vi "Upload File to Azure Container.vi"() -> ()   [LabVIEW 2015]
doc: "Demonstrates how to upload a file to an Azure Blob Service container."
uses:
  Core/Azure Credentials.ctl
  Blob Storage/Blob Type.ctl
  Core/NI_Azure_Core.lvlib
  Core/Session/Session.lvclass
  Blob Storage/NI_Azure_Blob.lvlib
panel:
  in  "File to Upload":path
  in  "Access Key":string
  in  "Storage Account Name":string
  in  "Destination Container":string
  # "Overview: Demonstrates how to upload a file to an Azure Blob Service container.\nRequirements: NI Cloud Toolkit for Azure and a registered Microsoft Azure account\nInstructions:\n1. Specify the Storage Account Name and Access Key for your Azure account. You can create an account at http://azure.microsoft.com.\n2. Specify a Destination Container for the file. If you have not created a container, you can run the Create New Azure Container.vi example to create a new container.\n3. Specify the File to Upload.\n4. Run the VI. The specified file will be placed in the specified container."
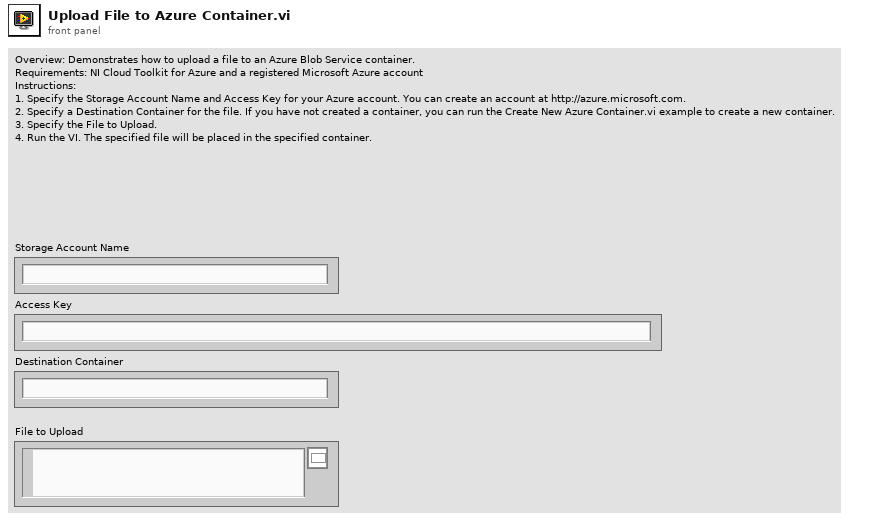
[diagram p1: front panel]
types:
  T1 = typedef "NI_Azure_Core.lvlib/Azure Credentials.ctl" = cluster{"Storage Account Name":string, "Access Key":string}
  T2 = typedef "NI_Azure_Blob.lvlib/Blob Type.ctl" = enum16{"BlockBlob", "PageBlob", "AppendBlob"}
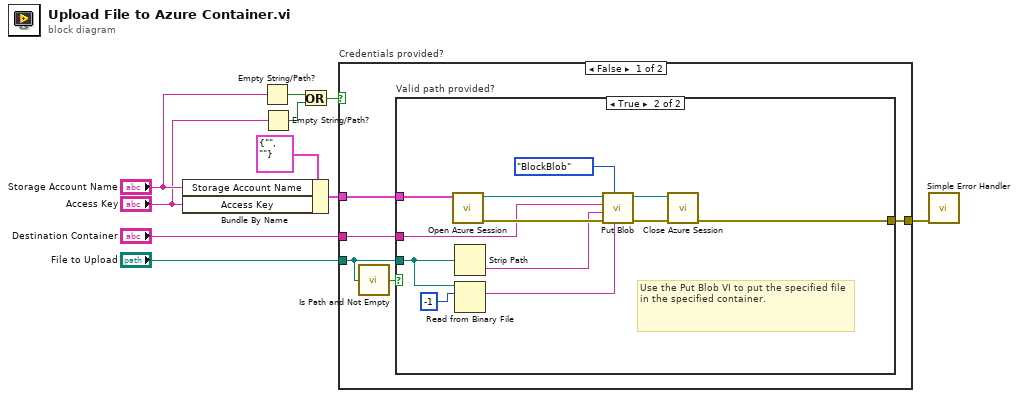
[diagram p0: block diagram]
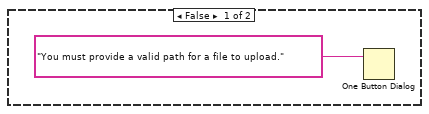
[diagram p2: hidden frame]
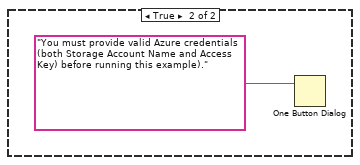
[diagram p3: hidden frame]
diagram:
  n1 = Bundle By Name(cluster=T1 {"Storage Account Name"="", "Access Key"=""} ("Credentials"), "Storage Account Name"="Storage Account Name", "Access Key"="Access Key") -> (w5:T1)
  n2 = Empty String/Path?(string/path="Storage Account Name") -> (empty?=w9:bool)
  n3 = Empty String/Path?(string/path="Access Key") -> (empty?=w10:bool)
  n4 = Or(x=w9, y=w10) -> (x .or. y?=w6:bool)
  n5 = case "Credentials provided?" shown="False" w6 {
    tunnel: w5 -> [w15 _]
    tunnel: "File to Upload" -> [w14 _]
    tunnel: "Destination Container" -> [w12 _]
    tunnel: [w11 _] -> w1
    frame False {
      n6 = call <vilib>:"Is Path and Not Empty.vi"("path"=w14) -> ("Is Path and Not Empty?"=w13:bool)  [unwired: 4 in]
      n7 = case "Valid path provided?" shown="True" w13 {
        tunnel: w15 -> [_ w28]
        tunnel: w14 -> [_ w24]
        tunnel: w12 -> [_ w19]
        tunnel: [_ w23] -> w11
        frame False {
          n8 = One Button Dialog(message="You must provide a valid path for a file to upload.") -> ()  [unwired: 1 in, 1 out]
        }
        frame True {
          # "Use the Put Blob VI to put the specified file in the specified container."
          n9 = call "Open Azure Session.vi"("Credentials"=w28) -> ("error out"=w27:errorcluster, "Azure Session"=w26:refnum<class "Session.lvclass">)  [unwired: 9 in]
          n10 = Strip Path(path=w24) -> (name=w18:string)  [unwired: 1 out]
          n11 = Read from Binary File(10:-1 ("count (1)"), 11:w24) -> (2:w21:string)  [unwired: 4 in, 3 out]
          n12 = call "Put Blob.vi"("Blob Content"=w21, "Blob type"=Blob_Type."BlockBlob", "error in (no error)"=w27, "Blob"=w18, "Container"=w19, "Azure Session in"=w26) -> ("error out"=w20:errorcluster, "Azure Session out"=w17:refnum<class "Session.lvclass">)  [unwired: 4 in]
          n13 = call "Close Azure Session.vi"("error in (no error)"=w20, "Azure Session"=w17) -> ("error out"=w23:errorcluster)  [unwired: 9 in]
        }
      }
    }
    frame True {
      n14 = One Button Dialog(message="You must provide valid Azure credentials (both Storage Account Name and Access Key) before running this example).") -> ()  [unwired: 1 in, 1 out]
    }
  }
  n15 = call <vilib>:"Simple Error Handler.vi"("error in (no error)"=w1) -> ()  [unwired: 4 in, 5 out]
